vi "ZM_state.vi"(6 "ZB":bool[](array[boolean])=[FALSE, FALSE], 9 "XB":bool[](array[boolean])=[FALSE, FALSE, FALSE, FALSE, FALSE], 10 "Z_In":cluster{"Z_Source":T1, "Z_State":T2}={"Z_Source"=enum."local disabled", "Z_State"=enum."alarm"}, 11 "ZM_state in":refnum<class "HE_ZM_state.lvclass">) -> (3 "ZM_state out":refnum<class "HE_ZM_state.lvclass">)   [LabVIEW 2019, in "Heating.lvlib" / "HE_ZM_state.lvclass"]
uses:
  HE_ZM_state.lvclass
  D:/my_projects/projects/Algorithms/Labview/19/Sequence/State/State.lvclass
  ctl/Z_source.ctl
  ctl/Z_State.ctl
  HE_ZM_state.lvclass/HE_ZM_state.ctl
  ctl/ZM_State.ctl
  Sequence/State/State.lvclass
  Heating.lvlib
panel:
  # "XB01 contactor on\nXB02 contactor off\nXB24 local hand on\nheating end\ncooling end"
  # "ZB01 contactor on reg\nZB02 contactor not off reg"
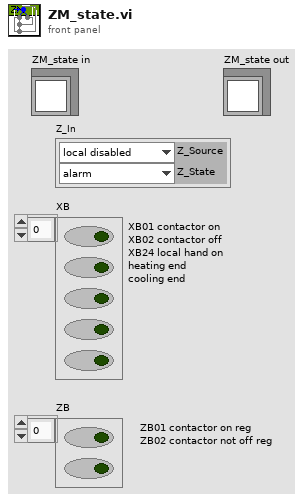
[diagram p1: front panel]
types:
  T1 = typedef "Heating.lvlib/Z_source.ctl" = enum8{"initialize", "local disabled", "local hand", "hand", "auto", "dist"}
  T2 = typedef "Heating.lvlib/Z_State.ctl" = enum8{"initialization", "alarm", "disabled", "not ready", "stop ready", "reserv", "switched off", "reserv2", "switched on", "check", "on min", "decrease out", "on", "increase out", "on max"}
  T3 = typedef "Heating.lvlib/ZM_State.ctl" = enum8{"initialization", "stop", "start_cmd", "contactor_on_cmd", "heating", "on", "stop_cmd", "power_down", "contactor_off_cmd", "cooling", "restart_delay"}
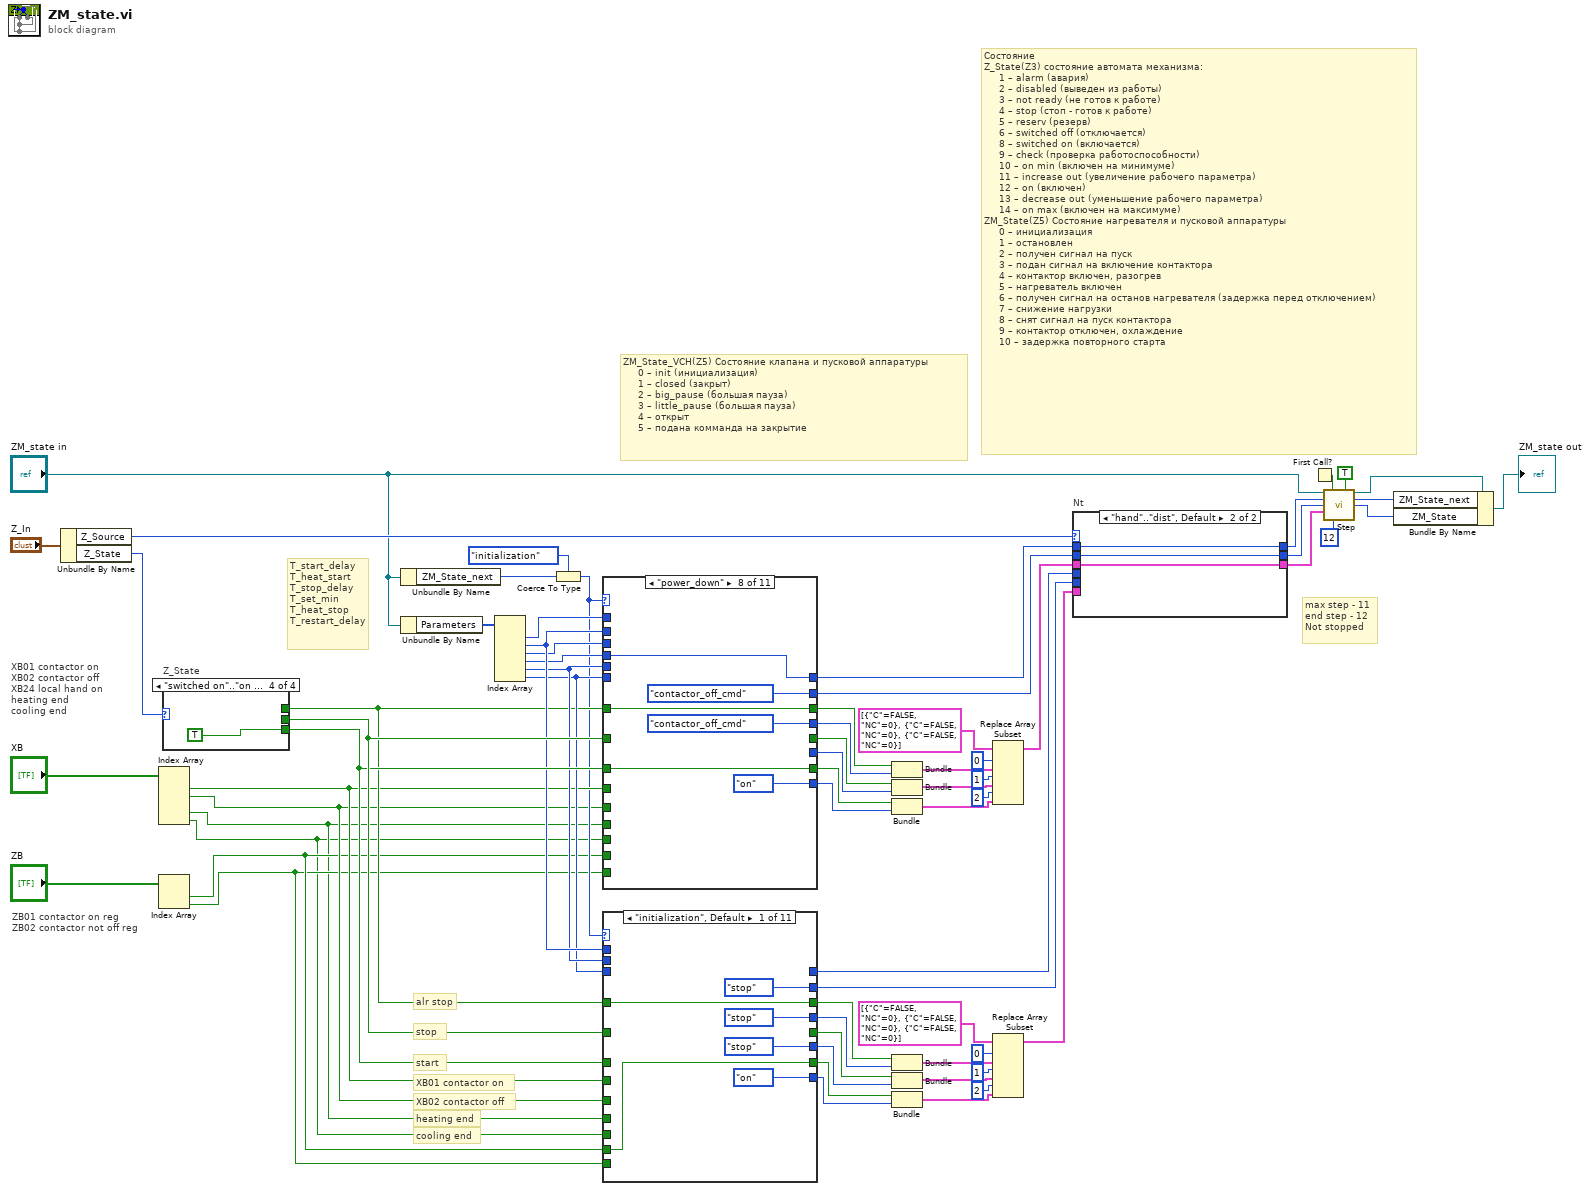
[diagram p0: block diagram]
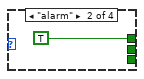
[diagram p3: hidden frame]
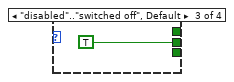
[diagram p4: hidden frame]
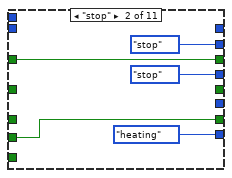
[diagram p5: hidden frame]
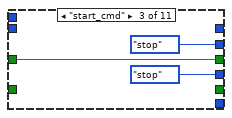
[diagram p6: hidden frame]
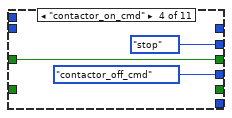
[diagram p7: hidden frame]
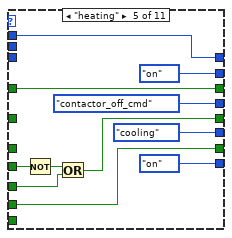
[diagram p8: hidden frame]
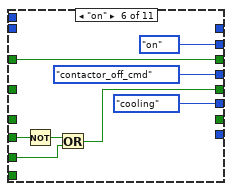
[diagram p9: hidden frame]
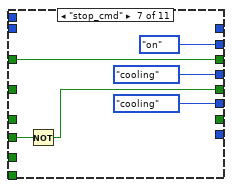
[diagram p10: hidden frame]
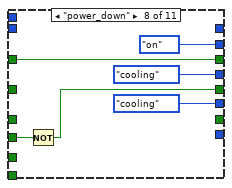
[diagram p11: hidden frame]
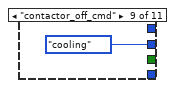
[diagram p12: hidden frame]
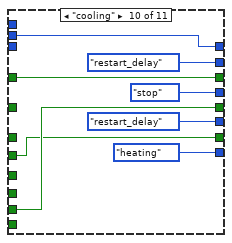
[diagram p13: hidden frame]
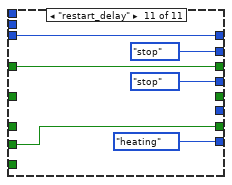
[diagram p14: hidden frame]
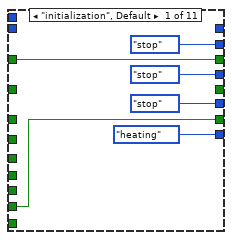
[diagram p15: hidden frame]
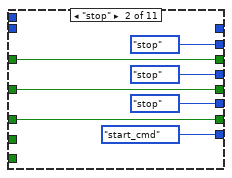
[diagram p16: hidden frame]
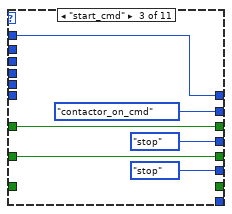
[diagram p17: hidden frame]
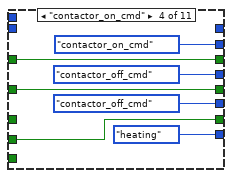
[diagram p18: hidden frame]
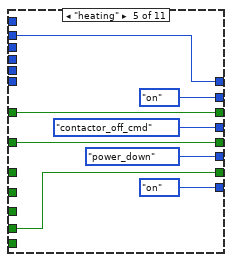
[diagram p19: hidden frame]
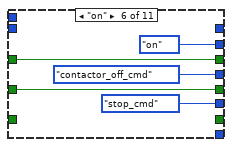
[diagram p20: hidden frame]
diagram:
  # "cooling end"
  # "heating end"
  # "XB02 contactor off"
  # "XB01 contactor on"
  # "alr stop"
  # "ZB01 contactor on reg\nZB02 contactor not off reg"
  # "XB01 contactor on\nXB02 contactor off\nXB24 local hand on\nheating end\ncooling end"
  # "T_start_delay\nT_heat_start\nT_stop_delay\nT_set_min\nT_heat_stop\nT_restart_delay"
  # "start"
  # "stop"
  # "Состояние\nZ_State(Z3) состояние автомата механизма:\n     1 – alarm (авария)\n     2 – disabled (выведен из работы)\n     3 – not ready (не готов к работе)\n     4 – stop (стоп - готов к работе)\n     5 – reserv (резерв)\n     6 – switched off (отключается)\n     8 – switched on (включается)\n     9 – check (проверка работоспособности)\n     10 – on min (включен на минимуме)\n     11 – increase out (увеличение рабочего параметра)\n     12 – on (включен)\n     13 – decrease out (уменьшение рабочего параметра)\n     14 – on max (включен на максимуме)\nZM_State(Z5) Состояние нагревателя и пусковой аппаратуры\n     0 – инициализация\n     1 – остановлен\n     2 – получен сигнал на пуск\n     3 – подан сигнал на включение контактора\n     4 – контактор включен, разогрев\n     5 – нагреватель включен\n     6 – получен сигнал на останов нагревателя (задержка перед отключением)\n     7 – снижение нагрузки\n     8 – снят сигнал на пуск контактора\n     9 – контактор отключен, охлаждение\n     10 – задержка повторного старта"
  # "ZM_State_VCH(Z5) Состояние клапана и пусковой аппаратуры\n     0 – init (инициализация)\n     1 – сlosed (закрыт)\n     2 – big_pause (большая пауза)\n     3 – little_pause (большая пауза)\n     4 – открыт\n     5 – подана комманда на закрытие"
  # "max step - 11\nend step - 12\nNot stopped"
  n1 = Unbundle By Name("Z_In") -> ("Z_Source"=w8:T1, "Z_State"=w45:T2)
  n2 = Index Array(array="XB") -> (element #1=w47:bool, element #2=w42:bool, element #4=w39:bool, element #5=w38:bool)  [unwired: 5 in, 1 out]
  n3 = Index Array(array="ZB") -> (element #1=w41:bool, element #2=w40:bool)  [unwired: 2 in]
  n4 = case "Z_State" shown="\"switched on\"..\"on max\"" w45 {
    tunnel: [_ _ TRUE _] -> w57
    tunnel: [_ _ _ TRUE] -> w56
    tunnel: [_ TRUE _ _] -> w49
    frame "initialization" {
    }
    frame "alarm" {
    }
    frame "disabled".."switched off", Default {
    }
    frame "switched on".."on max" {
    }
  }
  n5 = Unbundle By Name("ZM_state in") -> ("ZM_State_next"=w11:T3)
  n6 = Unbundle By Name("ZM_state in") -> ("Parameters"=w9:u32[])
  n7 = Index Array(array=w9) -> (element #1=w55:u32, element #2=w54:u32, element #3=w53:u32, element #4=w52:u32, element #5=w51:u32, element #6=w50:u32)  [unwired: 6 in]
  n8 = Coerce To Type(0:w11, 1:ZM_State."initialization" ("ZM_State")) -> (2:w43:T3)
  n9 = case shown="\"power_down\"" w43 {
    tunnel: [_ _ w88 _ w103 _ w113 w116 _ w136 w143] -> w7
    tunnel: [ZM_State."heating" ("ZM_State") ZM_State."start_cmd" ("ZM_State") _ ZM_State."heating" ("ZM_State") ZM_State."on" ("ZM_State") _ ZM_State."on" ("ZM_State") ZM_State."on" ("ZM_State") ZM_State."contactor_on_cmd" ("ZM_State") ZM_State."contactor_on_cmd" ("ZM_State") _] -> w26
    tunnel: [w75 w83 _ w94 w101 _ w114 w120 w132 w135 _] -> w27
    tunnel: [ZM_State."stop" ("ZM_State") ZM_State."stop" ("ZM_State") ZM_State."contactor_on_cmd" ("ZM_State") ZM_State."contactor_on_cmd" ("ZM_State") ZM_State."on" ("ZM_State") ZM_State."on" ("ZM_State") ZM_State."power_down" ("ZM_State") ZM_State."contactor_off_cmd" ("ZM_State") ZM_State."contactor_off_cmd" ("ZM_State") ZM_State."restart_delay" ("ZM_State") ZM_State."stop" ("ZM_State")] -> w6
    tunnel: w57 -> [_ w78 w89 w96 w104 w109 _ _ _ _ _]
    tunnel: w56 -> [_ w83 _ _ _ _ w114 w120 w132 w135 _]
    tunnel: w55 -> [_ _ w88 _ _ _ _ _ _ _ _]
    tunnel: [_ w78 w89 w96 w104 w109 _ _ w126 w134 _] -> w29
    tunnel: [ZM_State."stop" ("ZM_State") ZM_State."stop" ("ZM_State") ZM_State."stop" ("ZM_State") ZM_State."contactor_off_cmd" ("ZM_State") ZM_State."power_down" ("ZM_State") ZM_State."stop_cmd" ("ZM_State") _ _ ZM_State."cooling" ("ZM_State") ZM_State."restart_delay" ("ZM_State") _] -> w28
    tunnel: w47 -> [_ _ _ w94 _ _ _ _ w130 _ _]
    tunnel: w54 -> [_ _ _ _ w103 _ _ _ _ _ _]
    tunnel: w49 -> [w76 w82 w87 w95 w102 w108 w115 w121 w128 w140 w144]
    tunnel: [w76 w82 w87 w95 w102 w108 w115 w121 w127 w140 w144] -> w34
    tunnel: [ZM_State."stop" ("ZM_State") ZM_State."stop" ("ZM_State") ZM_State."stop" ("ZM_State") ZM_State."contactor_off_cmd" ("ZM_State") ZM_State."contactor_off_cmd" ("ZM_State") ZM_State."contactor_off_cmd" ("ZM_State") ZM_State."contactor_off_cmd" ("ZM_State") ZM_State."contactor_off_cmd" ("ZM_State") ZM_State."stop" ("ZM_State") ZM_State."stop" ("ZM_State") ZM_State."stop" ("ZM_State")] -> w33
    tunnel: w53 -> [_ _ _ _ _ _ w113 _ _ _ _]
    tunnel: w52 -> [_ _ _ _ _ _ _ w116 _ _ _]
    tunnel: w42 -> [_ _ _ _ _ _ _ _ w129 _ _]
    tunnel: w51 -> [_ _ _ _ _ _ _ _ _ w136 _]
    tunnel: w50 -> [_ _ _ _ _ _ _ _ _ _ w143]
    tunnel: w41 -> [w75 _ _ _ _ _ _ _ _ _ _]
    tunnel: w40 -> [_ _ _ _ _ _ _ _ _ _ _]
    tunnel: w39 -> [_ _ _ _ w101 _ _ _ _ _ _]
    tunnel: w38 -> [_ _ _ _ _ _ _ _ _ w134 _]
    frame "initialization", Default {
    }
    frame "stop" {
    }
    frame "start_cmd" {
    }
    frame "contactor_on_cmd" {
    }
    frame "heating" {
    }
    frame "on" {
    }
    frame "stop_cmd" {
    }
    frame "power_down" {
    }
    frame "contactor_off_cmd" {
      n10 = Not(x=w130) -> (.not. x?=w131:bool)
      n11 = Or(x=w131, y=w129) -> (x .or. y?=w126:bool)
      n12 = And(x=w128, y=w126) -> (x .and. y?=w127:bool)
    }
    frame "cooling" {
    }
    frame "restart_delay" {
    }
  }
  n13 = case shown="\"initialization\", Default" w43 {
    tunnel: [_ _ _ _ w172 _ _ _ _ w197 w206] -> w3
    tunnel: [ZM_State."on" ("ZM_State") ZM_State."heating" ("ZM_State") _ _ ZM_State."on" ("ZM_State") _ _ _ _ ZM_State."heating" ("ZM_State") ZM_State."heating" ("ZM_State")] -> w12
    tunnel: [w149 w154 _ _ w162 _ _ _ _ w194 w205] -> w13
    tunnel: [ZM_State."stop" ("ZM_State") ZM_State."stop" ("ZM_State") ZM_State."stop" ("ZM_State") ZM_State."stop" ("ZM_State") ZM_State."on" ("ZM_State") ZM_State."on" ("ZM_State") ZM_State."on" ("ZM_State") ZM_State."on" ("ZM_State") ZM_State."cooling" ("ZM_State") ZM_State."restart_delay" ("ZM_State") ZM_State."stop" ("ZM_State")] -> w2
    tunnel: w57 -> [_ _ _ _ _ _ _ _ _ _ _]
    tunnel: w56 -> [_ _ _ _ _ _ _ _ _ _ _]
    tunnel: [_ _ _ _ w163 w173 w184 w190 _ w195 _] -> w15
    tunnel: [ZM_State."stop" ("ZM_State") _ _ _ ZM_State."cooling" ("ZM_State") ZM_State."cooling" ("ZM_State") ZM_State."cooling" ("ZM_State") ZM_State."cooling" ("ZM_State") _ ZM_State."restart_delay" ("ZM_State") _] -> w14
    tunnel: w47 -> [_ w154 _ _ w165 w175 w185 w191 _ w194 w205]
    tunnel: w54 -> [_ _ _ _ w172 _ _ _ _ _ _]
    tunnel: w49 -> [w150 w155 w158 w161 w171 w180 w186 w192 _ w196 w207]
    tunnel: [w150 w155 w158 w161 w171 w180 w186 w192 _ w196 w207] -> w17
    tunnel: [ZM_State."stop" ("ZM_State") ZM_State."stop" ("ZM_State") ZM_State."stop" ("ZM_State") ZM_State."contactor_off_cmd" ("ZM_State") ZM_State."contactor_off_cmd" ("ZM_State") ZM_State."contactor_off_cmd" ("ZM_State") ZM_State."cooling" ("ZM_State") ZM_State."cooling" ("ZM_State") _ ZM_State."stop" ("ZM_State") ZM_State."stop" ("ZM_State")] -> w16
    tunnel: w42 -> [_ _ _ _ w164 w174 _ _ _ _ _]
    tunnel: w51 -> [_ _ _ _ _ _ _ _ _ w197 _]
    tunnel: w50 -> [_ _ _ _ _ _ _ _ _ _ w206]
    tunnel: w41 -> [w149 _ _ _ _ _ _ _ _ _ _]
    tunnel: w40 -> [_ _ _ _ _ _ _ _ _ _ _]
    tunnel: w39 -> [_ _ _ _ w162 _ _ _ _ _ _]
    tunnel: w38 -> [_ _ _ _ _ _ _ _ _ w195 _]
    frame "initialization", Default {
    }
    frame "stop" {
    }
    frame "start_cmd" {
    }
    frame "contactor_on_cmd" {
    }
    frame "heating" {
      n14 = Not(x=w165) -> (.not. x?=w166:bool)
      n15 = Or(x=w166, y=w164) -> (x .or. y?=w163:bool)
    }
    frame "on" {
      n16 = Not(x=w175) -> (.not. x?=w176:bool)
      n17 = Or(x=w176, y=w174) -> (x .or. y?=w173:bool)
    }
    frame "stop_cmd" {
      n18 = Not(x=w185) -> (.not. x?=w184:bool)
    }
    frame "power_down" {
      n19 = Not(x=w191) -> (.not. x?=w190:bool)
    }
    frame "contactor_off_cmd" {
    }
    frame "cooling" {
    }
    frame "restart_delay" {
    }
  }
  n20 = Bundle(w34, "ZM_State"=w33) -> (w35:cluster{bool, "ZM_State":T3})  [unwired: 1 in]
  n21 = Bundle("XB"=w29, "ZM_State"=w28) -> (w30:cluster{"XB":bool, "ZM_State":T3})  [unwired: 1 in]
  n22 = Bundle("XB"=w27, "ZM_State"=w26) -> (w25:cluster{"XB":bool, "ZM_State":T3})  [unwired: 1 in]
  n23 = Bundle(w17, "ZM_State"=w16) -> (w20:cluster{bool, "ZM_State":T3})  [unwired: 1 in]
  n24 = Bundle("XB"=w15, "ZM_State"=w14) -> (w23:cluster{"XB":bool, "ZM_State":T3})  [unwired: 1 in]
  n25 = Bundle("XB"=w13, "ZM_State"=w12) -> (w24:cluster{"XB":bool, "ZM_State":T3})  [unwired: 1 in]
  n26 = Replace Array Subset(array=cluster{"C":bool, "NC":u32}[] [{"C"=FALSE, "NC"=0}, {"C"=FALSE, "NC"=0}, {"C"=FALSE, "NC"=0}] ("appended array"), new element #1=w35, index #1=0 ("index"), new element #2=w30, index #2=1 ("index"), new element #3=w25, index #3=2 ("index")) -> (w5:cluster{"C":bool, "NC":u32}[])
  n27 = Replace Array Subset(array=cluster{"C":bool, "NC":u32}[] [{"C"=FALSE, "NC"=0}, {"C"=FALSE, "NC"=0}, {"C"=FALSE, "NC"=0}] ("appended array"), new element #1=w20, index #1=0 ("index"), new element #2=w23, index #2=1 ("index"), new element #3=w24, index #3=2 ("index")) -> (w4:cluster{"C":bool, "NC":u32}[])
  n28 = case "Nt" shown="\"hand\"..\"dist\", Default" w8 {
    tunnel: w6 -> [_ w213]
    tunnel: w5 -> [_ w212]
    tunnel: [w209 w213] -> w65
    tunnel: [w210 w212] -> w64
    tunnel: w2 -> [w209 _]
    tunnel: w4 -> [w210 _]
    tunnel: w3 -> [w208 _]
    tunnel: [w208 w211] -> w66
    tunnel: w7 -> [_ w211]
    frame "local disabled", "local hand" {
    }
    frame "hand".."dist", Default {
    }
  }
  n29 = First Call?() -> (First Call?: T/F=w67:bool)
  n30 = call "Step.vi"("State in"="ZM_state in", "Reset"=w67, "Start in"=TRUE ("Start"), "t"=w66, "Nt"=w65, "C_table"=w64, "N end step"=u32 12) -> ("State out"=w58:refnum<class "HE_ZM_state.lvclass">, "N next"=w61:u32, "N curr"=w62:u32)  [unwired: 5 in, 1 out]
  n31 = Bundle By Name(cluster=w58, "ZM_State_next"=w61, "ZM_State"=w62) -> (→"ZM_state out":refnum<class "HE_ZM_state.lvclass">)
